vi "getGlyphFile.vi"(8 "error in (no error)":errorcluster, 11 "DMA_Write in":refnum<class "DMA_Write.lvclass">) -> (0 "error out":errorcluster, 2 "Glyph File":string, 3 "DMA_Write out":refnum<class "DMA_Write.lvclass">)   [LabVIEW 2013, in "DMA_Write.lvclass"]
doc: "Dynamic Dispatch VI. Returns the name of the glyph file to be used as a glyph in the tree control. A empty string means no glyph."
uses:
  DMA_Write.lvclass
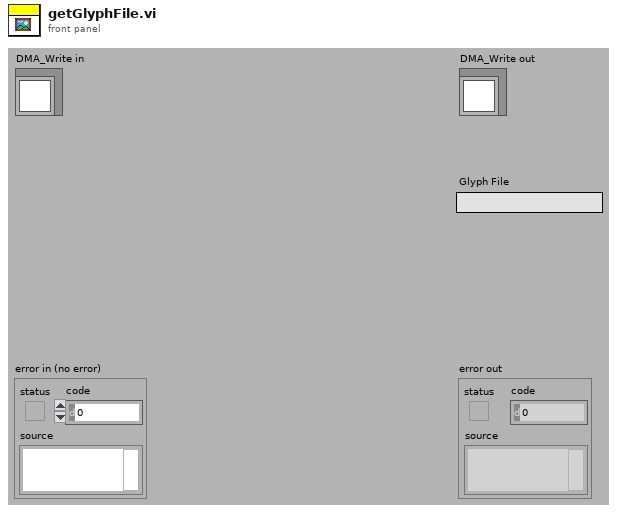
[diagram p1: front panel]
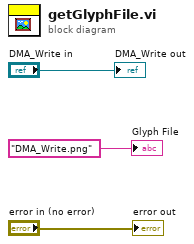
[diagram p0: block diagram]
diagram:
  "error out" <- "error in (no error)"
  "DMA_Write out" <- "DMA_Write in"
  "Glyph File" <- "DMA_Write.png" ("Glyph File")
